vi "Irregular Array Subset (bool).vi"(8 "Mask":bool[](array[boolean]), 10 "Array":bool[](array[boolean])) -> (0 "Indices":i32[](array[numeric]), 2 "Array Subset":bool[](array[boolean]))   [LabVIEW 2020]
doc: "Extracts the values from the input array for which the corresponding boolean inputs are TRUE."
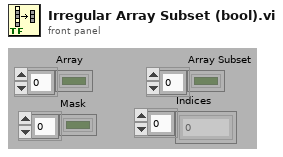
[diagram p1: front panel]
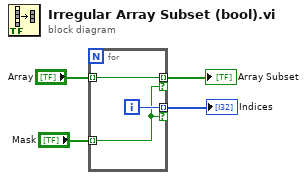
[diagram p0: block diagram]
diagram:
  n1 = for {
    tunnel: "Mask" -> [w5] mode=indexing
    tunnel: "Array" -> [w7] mode=indexing
    tunnel: [w7] -> w2 mode=indexing if=w5
    tunnel: [w6] -> w1 mode=indexing if=w5
    i -> [w6]
  }
  "Indices" <- w1
  "Array Subset" <- w2
